vi "Write Task Hierarchy.vi"(8 "error in (no error)":errorcluster, 10 "Task Hierarchy":i64=-1, 11 "Composite Map Task in":refnum<class "Composite ID-Map Task.lvclass">) -> (0 "error out":errorcluster, 3 "Composite Map Task out":refnum<class "Composite ID-Map Task.lvclass">)   [LabVIEW 2024, in "Composite ID-Map Task.lvclass"]
uses:
  Composite ID-Map Task.lvclass
  Composite ID-Map Task.lvclass/Composite ID-Map Task.ctl
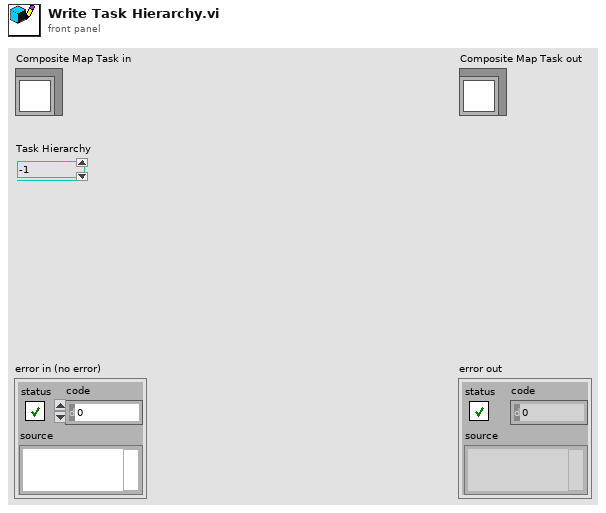
[diagram p1: front panel]
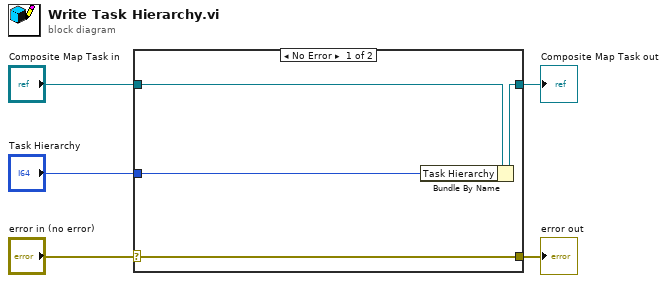
[diagram p0: block diagram]
diagram:
  n1 = case shown="No Error" "error in (no error)" {
    selector: "error in (no error)" -> [w9 w10]
    tunnel: [w9 w10] -> w4
    tunnel: [w7 w11] -> w2
    tunnel: "Composite Map Task in" -> [w8 w11]
    tunnel: "Task Hierarchy" -> [w6 _]
    frame No Error {
      n2 = Bundle By Name(cluster=w8, "Task Hierarchy"=w6) -> (w7:refnum<class "Composite ID-Map Task.lvclass">)
    }
    frame Error {
    }
  }
  "error out" <- w4
  "Composite Map Task out" <- w2
